vi "PAN_TCPSERVER_StartServerInstance.vi"(4 "client params":string, 5 "open panel":bool, 6 "max instances":i8=10, 7 "ID":string, 8 "error in (no error)":errorcluster, 9 "messages from sock Q":refnum<queue>, 10 "notifier In":refnum<notifier>, 11 "sock ID":refnum<k5>) -> (0 "error out":errorcluster)   [LabVIEW 2016]
uses:
  PAN_TCPSERVER_MsgStruct.ctl
panel:
  in  "VI Refnum":refnum<vi>
  in  "vi path":path
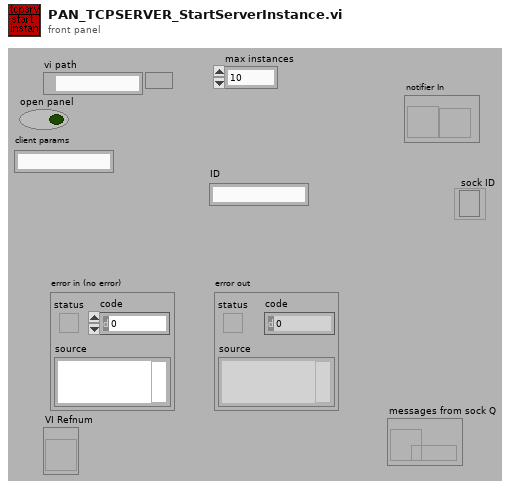
[diagram p1: front panel]
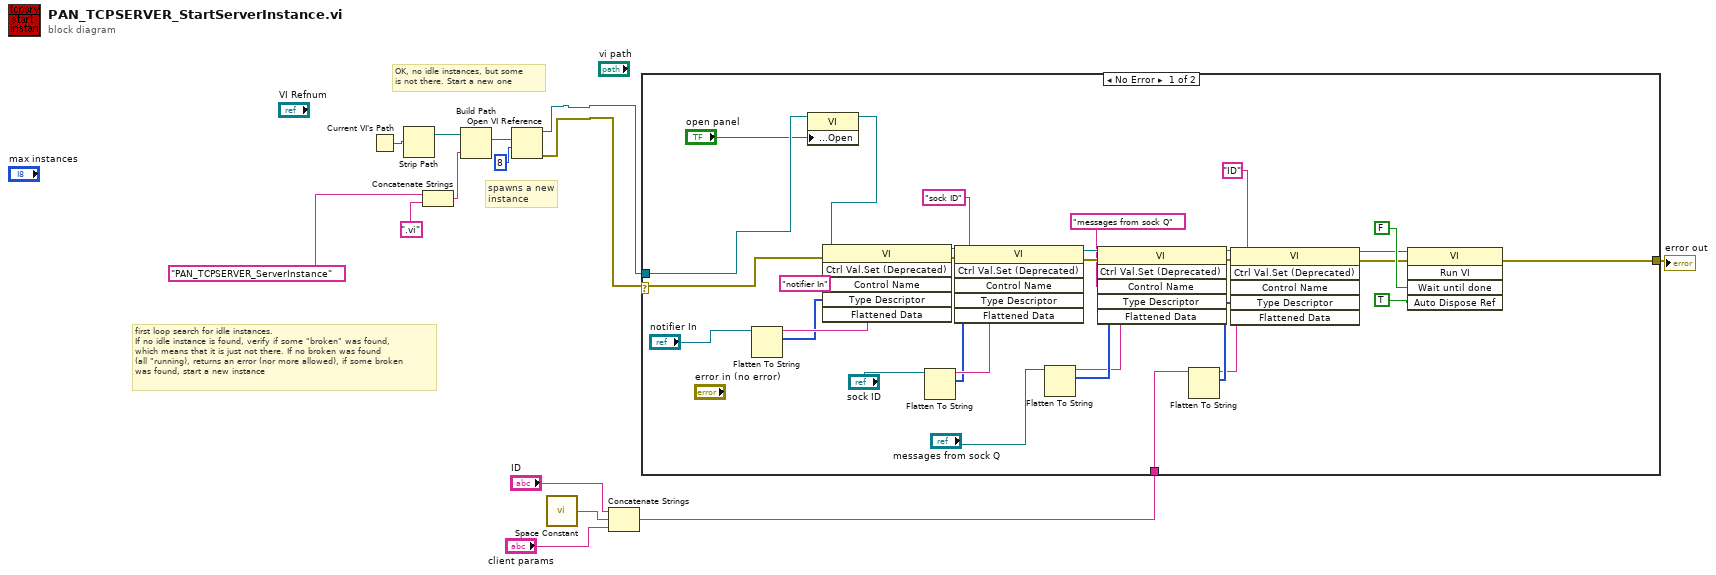
[diagram p0: block diagram]
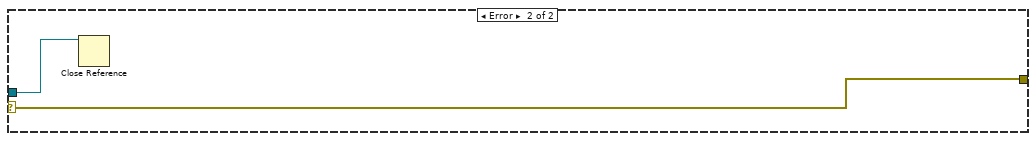
[diagram p2: hidden frame]
diagram:
  # "spawns a new\ninstance"
  # "OK, no idle instances, but some\nis not there. Start a new one"
  # "first loop search for idle instances.\nIf no idle instance is found, verify if some \"broken\" was found,\nwhich means that it is just not there. If no broken was found\n(all \"running), returns an error (nor more allowed), if some broken\nwas found, start a new instance"
  n1 = Current VI's Path() -> (path=w10:path)
  n2 = Strip Path(path=w10) -> (stripped path=w9:path)  [unwired: 1 out]
  n3 = Concatenate Strings("PAN_TCPSERVER_ServerInstance" ("name or relative path"), ".vi" ("string")) -> (w7:string)
  n4 = Build Path(base path=w9, name or relative path=w7) -> (appended path=w6:path)
  n5 = Open VI Reference(vi path=w6, options=8) -> (vi reference=w12:refnum<vi>, error out=w13:errorcluster)  [unwired: 1 in, 3 out]
  n6 = call <vilib>:"Space Constant.vi"() -> ("String"=w2:string)
  n7 = Concatenate Strings("ID", w2, "client params") -> (w3:string)
  n8 = case shown="No Error" w13 {
    selector: w13 -> [w20 w47]
    tunnel: [w25 w47] -> w14
    tunnel: w3 -> [w23 _]
    tunnel: w12 -> [w21 w46]
    frame No Error {
      n9 = Flatten To String(anything="notifier In") -> (data string=w43:string, type string=w42:i16[])  [unwired: 1 in, 3 out]
      n10 = property class="VI"(reference=w21, "Front Panel Window:Open"="open panel") -> (reference out=w22:refnum<vi>)  [unwired: 1 in, 1 out]
      n11 = invoke class="VI" method="Ctrl Val.Set (Deprecated)"(reference=w22, error in=w20, "Control Name"="notifier In", "Type Descriptor"=w42, "Flattened Data"=w43) -> (reference out=w41:refnum<vi>, error out=w40:errorcluster)  [unwired: 1 in, 4 out]
      n12 = Flatten To String(anything="sock ID") -> (data string=w37:string, type string=w36:i16[])  [unwired: 1 in, 3 out]
      n13 = invoke class="VI" method="Ctrl Val.Set (Deprecated)"(reference=w41, error in=w40, "Control Name"="sock ID", "Type Descriptor"=w36, "Flattened Data"=w37) -> (reference out=w35:refnum<vi>, error out=w34:errorcluster)  [unwired: 1 in, 4 out]
      n14 = Flatten To String(anything="messages from sock Q") -> (data string=w31:string, type string=w32:i16[])  [unwired: 1 in, 3 out]
      n15 = invoke class="VI" method="Ctrl Val.Set (Deprecated)"(reference=w35, error in=w34, "Control Name"="messages from sock Q", "Type Descriptor"=w32, "Flattened Data"=w31) -> (reference out=w30:refnum<vi>, error out=w29:errorcluster)  [unwired: 1 in, 4 out]
      n16 = Flatten To String(anything=w23) -> (data string=w26:string, type string=w27:i16[])  [unwired: 1 in, 3 out]
      n17 = invoke class="VI" method="Ctrl Val.Set (Deprecated)"(reference=w30, error in=w29, "Control Name"="ID", "Type Descriptor"=w27, "Flattened Data"=w26) -> (reference out=w16:refnum<vi>, error out=w15:errorcluster)  [unwired: 1 in, 4 out]
      n18 = invoke class="VI" method="Run VI"(reference=w16, error in=w15, "Wait until done"=FALSE, "Auto Dispose Ref"=TRUE ("Auto Dispose Reference")) -> (error out=w25:errorcluster)  [unwired: 1 in, 4 out]
    }
    frame Error {
      n19 = Close Reference(reference=w46) -> ()  [unwired: 1 in, 1 out]
    }
  }
  "error out" <- w14
